vi "To Pythonic - String Array.vi"(4 "String Array":string[](array[string])) -> (1 "Pythonic Value":string)   [LabVIEW 2016, in "OPI.lvclass"]
doc: "Convert LabVIEW data into valid pythonic representation."
uses:
  OPI.lvclass
  <vilib>/AdvancedString/Join Strings.vi
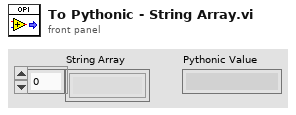
[diagram p1: front panel]
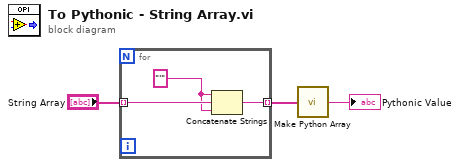
[diagram p0: block diagram]
diagram:
  n1 = for {
    tunnel: "String Array" -> [w6] mode=indexing
    tunnel: [w5] -> w3 mode=indexing
    w4 = "'" ("string")
    n2 = Concatenate Strings(w4, w6, w4) -> (w5:string)
  }
  n3 = call "Make Python Array.vi"("Pythonic Values"=w3) -> ("Pythonic Array"=→"Pythonic Value":string)
